vi "MALT HexStringToASCIIString.vi"(3 "string in":string="32 39 33 41 30 38 30 37 30 52") -> (1 "string out":string="293A08070R")   [LabVIEW 2018, in "AltonTech MALT200817.lvlib"]
uses:
  AltonTech MALT200817.lvlib
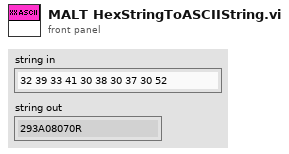
[diagram p1: front panel]
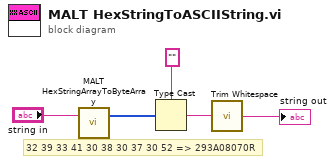
[diagram p0: block diagram]
diagram:
  # "32 39 33 41 30 38 30 37 30 52 => 293A08070R"
  n1 = call "MALT HexStringArrayToByteArray.vi"("HexStirngArray"="string in") -> ("ByteArrayOut"=w3:u8[])  [unwired: 2 in]
  n2 = Type Cast(type="", x=w3) -> (*(type *) &x=w2:string)
  n3 = call <vilib>:"Trim Whitespace.vi"("string"=w2) -> ("trimmed string"=→"string out":string)  [unwired: 1 in]
